vi "Register Request.vi"(8 "error in (no error)":errorcluster, 10 "Notifier":refnum<notifier>, 11 "OBS in":refnum<class "OBS.lvclass">) -> (0 "error out":errorcluster, 2 "Request ID":string, 3 "OBS out":refnum<class "OBS.lvclass">)   [LabVIEW 2022 SP3, in "obs-websocket-lv.lvlib" / "OBS.lvclass"]
uses:
  OBS.lvclass
  OBS.lvclass/OBS.ctl
  Response/Response.lvclass
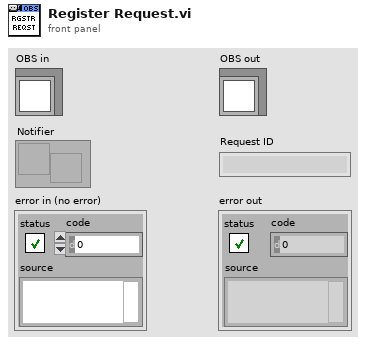
[diagram p1: front panel]
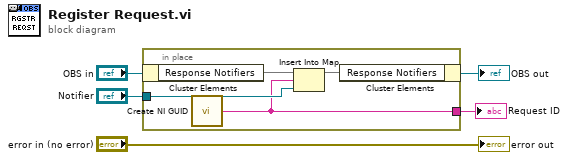
[diagram p0: block diagram]
diagram:
  n1 = in-place {
    in-place-border: "Notifier" -> [w8]
    in-place-border: [w6] -> w2
    n2 = in-place-cluster #1("OBS in") -> ("Response Notifiers"=w9:map{string, refnum<notifier>})
    n3 = call <vilib>:"Create NI GUID.vi"() -> ("NI GUID"=w6:string)
    n4 = Insert Into Map(map in=w9, key=w6, value=w8) -> (map out=w7:map{string, refnum<notifier>})  [unwired: 2 out]
    n5 = in-place-cluster #1("Response Notifiers"=w7) -> (→"OBS out":refnum<class "OBS.lvclass">)
  }
  "Request ID" <- w2
  "error out" <- "error in (no error)"
